vi "Transfer Sample.vi"(8 "error in (no error)":errorcluster, 11 "cRIO-CO2 in":refnum<class "cRIO-CO2.lvclass">) -> (0 "error out":errorcluster, 3 "cRIO-CO2 out":refnum<class "cRIO-CO2.lvclass">)   [LabVIEW 2015, in "cRIO-Carbondioxide.lvlib" / "cRIO-CO2.lvlib" / "cRIO-CO2.lvclass"]
uses:
  cRIO-CO2.lvclass
  cRIO-CO2.lvclass/cRIO-CO2.ctl
  <vilib>/ActorFramework/Time-Delayed Send Message/Time-Delay Override Options.ctl
  Controls/Sample Transfer State Enumerator.ctl
  subs/Sample/Sample.lvclass
  <vilib>/ActorFramework/Message Enqueuer/Message Enqueuer.lvclass/Message Enqueuer.ctl
  subs/Sample/Sample.lvclass/Sample.ctl
  Controls/Sample Transfer Container Enumerator.ctl
  Controls/Vacuum State Enumerator.ctl
  <vilib>/ActorFramework/Message Enqueuer/Enqueue.vi
  State Elapsed Time.vi
  <vilib>/ActorFramework/Message Priority Queue/Priority Enqueue.vi
  Transfer Line Messages/Sample Out Msg/Sample Out Msg.lvclass
panel:
  out "Waveform Chart":ext(graph)
  out "time stamp":timestamp
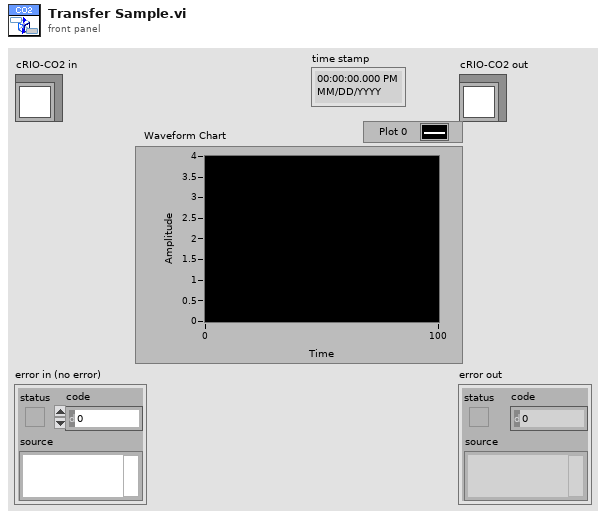
[diagram p1: front panel]
types:
  T1 = typedef "Time-Delay Override Options.ctl" = enum16{"Send next copy now", "Skip next scheduled copy", "Send next copy now and stop all further copies", "Stop all further copies"}
  T2 = typedef "Sample Transfer State Enumerator.ctl" = enum16{"Idle", "Initialize", "Check Containers", "Check Temperatures", "Start Turbo", "Warm Up Containers", "Prepare for purging", "Purge Capillary", "Purge", "Open Containers", "Introduce Sample", "Measure Base Pressure", "Home Syringe", "Start Freezer", "Freeze Target", "Crystalize", "Initiate Stash", "Stash", "Polish", "Stop Freezers", "Push Sample", "Complete", "Abort", "Error", "Undefined"}
  T3 = typedef "Sample Transfer Container Enumerator.ctl" = enum16{"None", "Sample 1", "Sample 2", "Sample 3", "Sample 4", "Sample 5", "Storage 01", "Storage 02", "Storage 03", "Storage 04", "Storage 05", "Storage 06", "Storage 07", "Storage 08", "Storage 09", "Storage 10", "Storage 11", "Storage 12", "Syringe", "Undefined"}
  T4 = typedef "Vacuum State Enumerator.ctl" = enum16{"Pressure Rising", "Plateau", "Pressure Dropping", "Valley", "Low Valley", "Leak", "Unknown"}
  T5 = typedef "cRIO-Carbondioxide.lvlib/cRIO-CO2.lvlib/cRIO-CO2.lvclass/Blowers Heaters Enumerator.ctl" = enum16{"Tank Blower 1", "Tank Blower 2", "Tank Blower 3", "Tank Blower 4", "Syringe Blower", "Syringe Heater", "Piston Heater", "Undefined"}
  T6 = typedef "Sample Container.ctl" = cluster{"Sample In":refnum<k21>, "Sample Name":refnum<k21>, "Ti Cathode":refnum<k21>, "SampleQ":refnum<queue>}
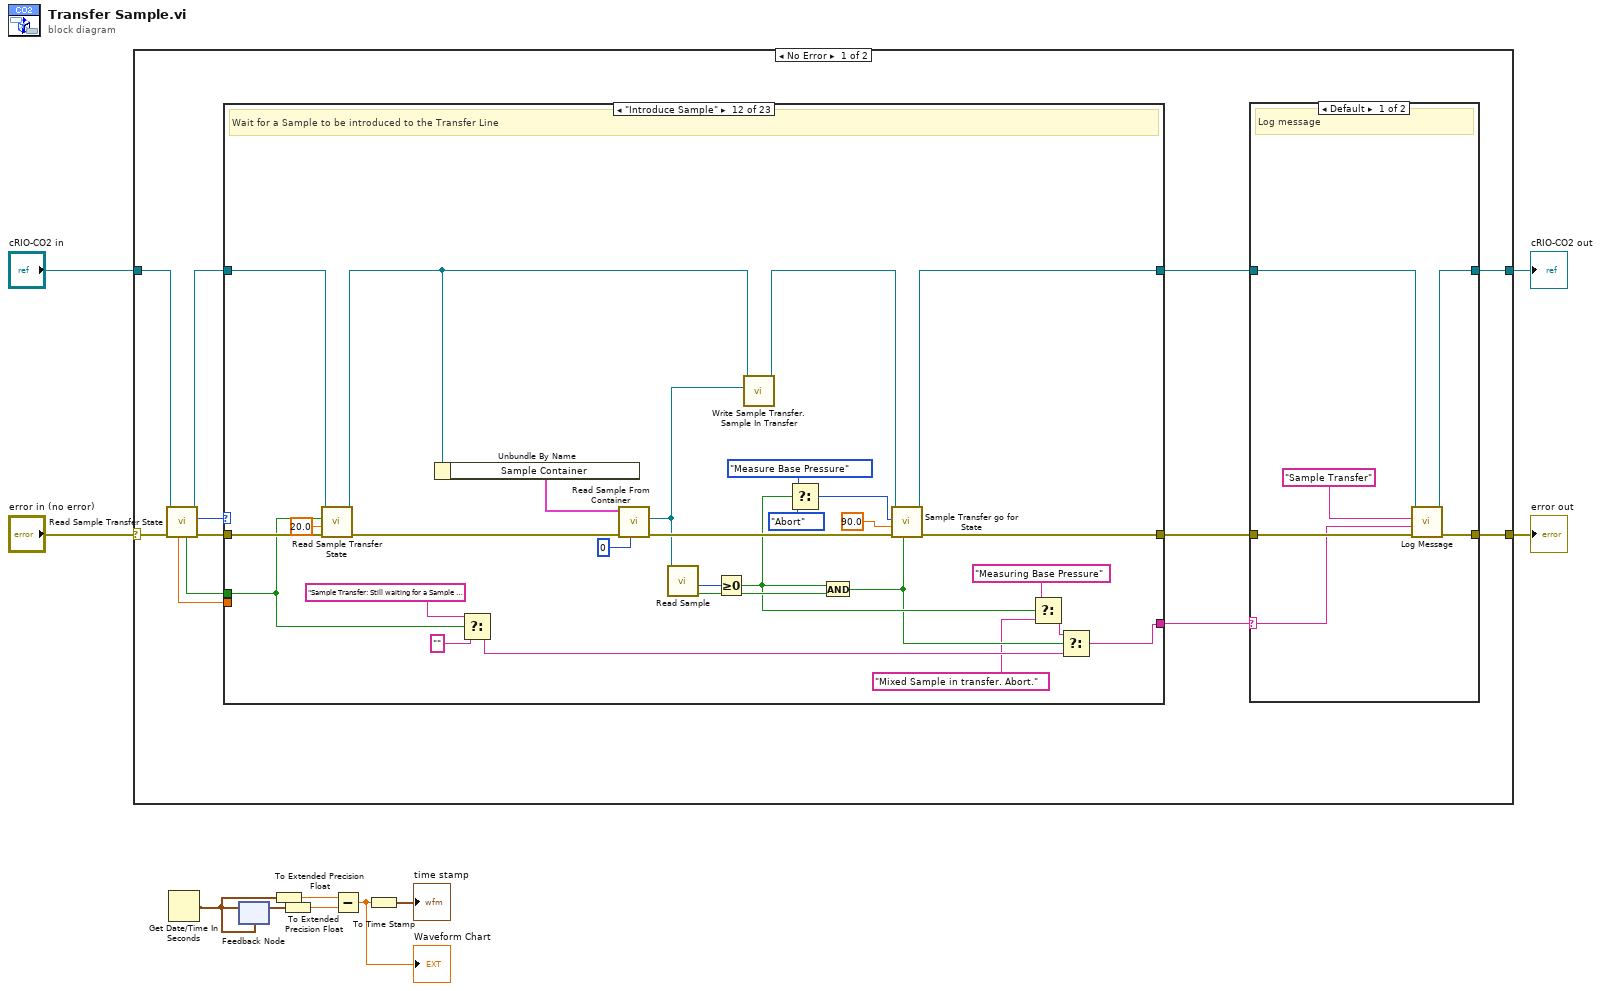
[diagram p0: block diagram]
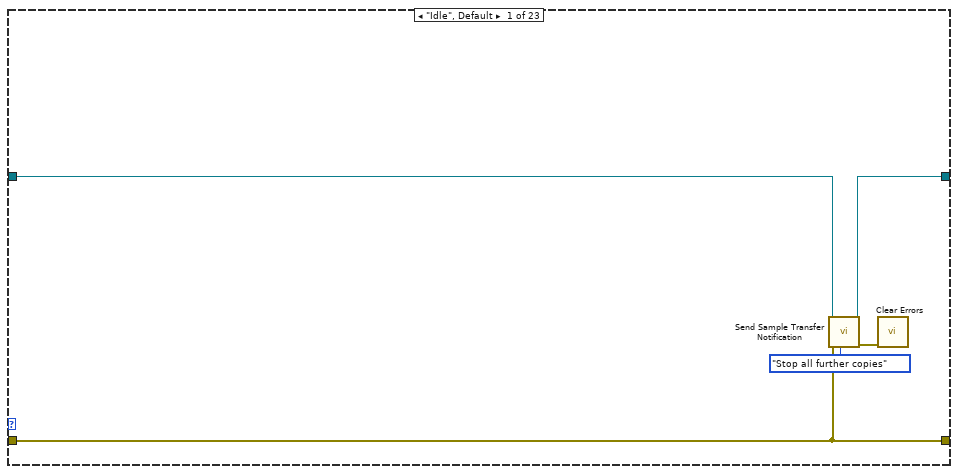
[diagram p3: hidden frame]
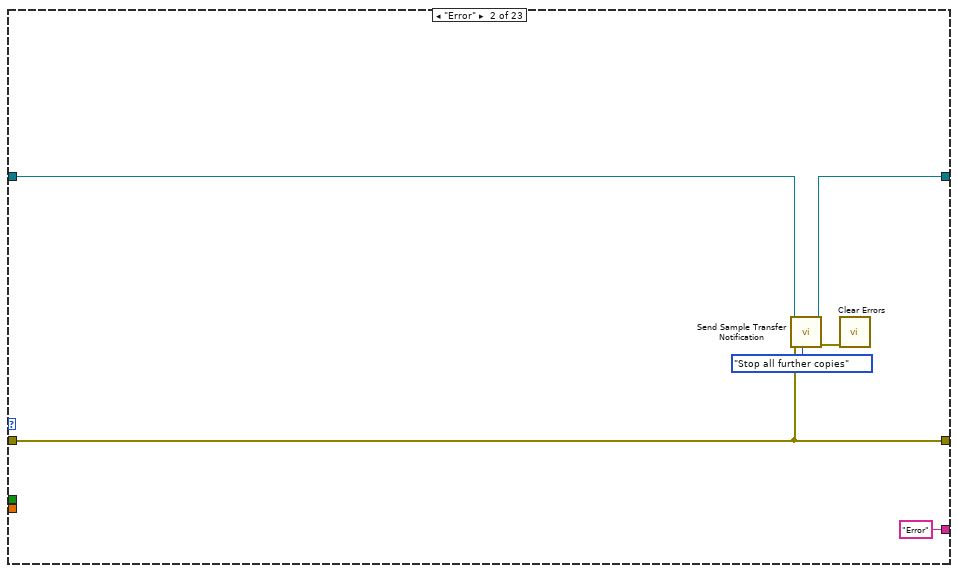
[diagram p4: hidden frame]
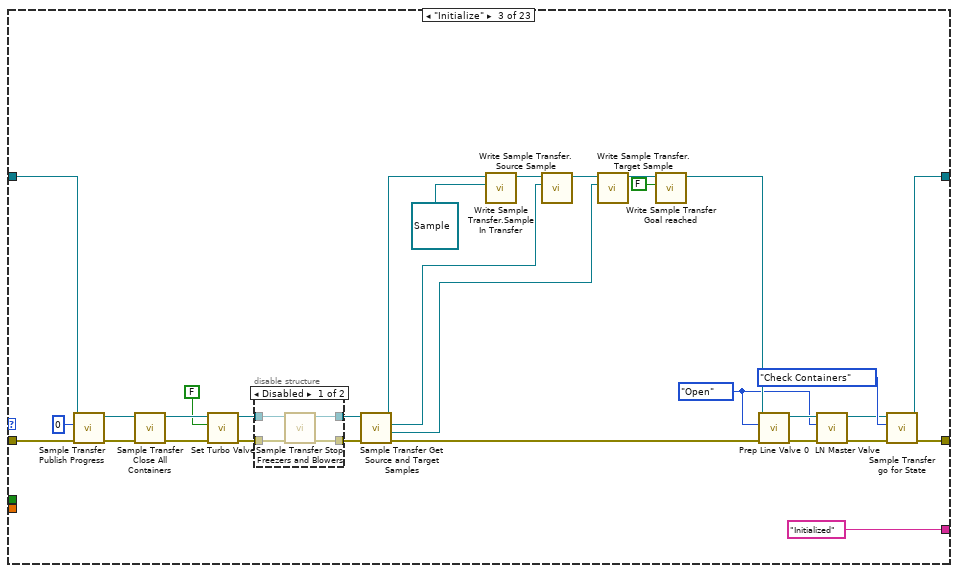
[diagram p5: hidden frame]
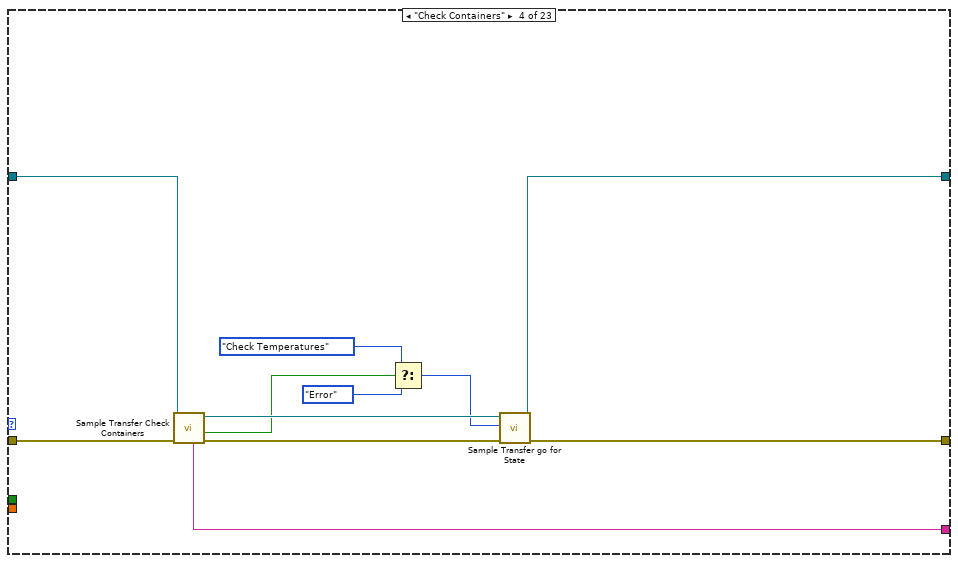
[diagram p7: hidden frame]
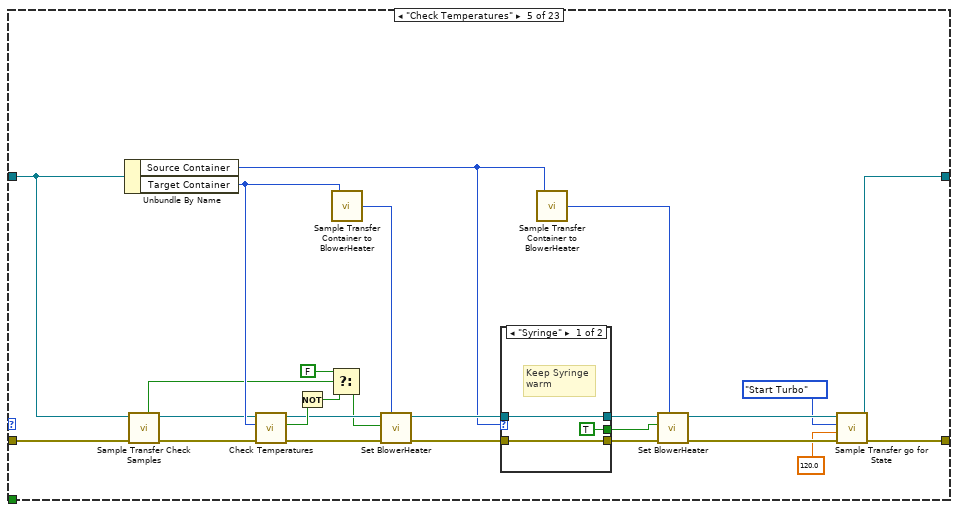
[diagram p8: hidden frame]
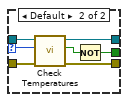
[diagram p9: hidden frame]
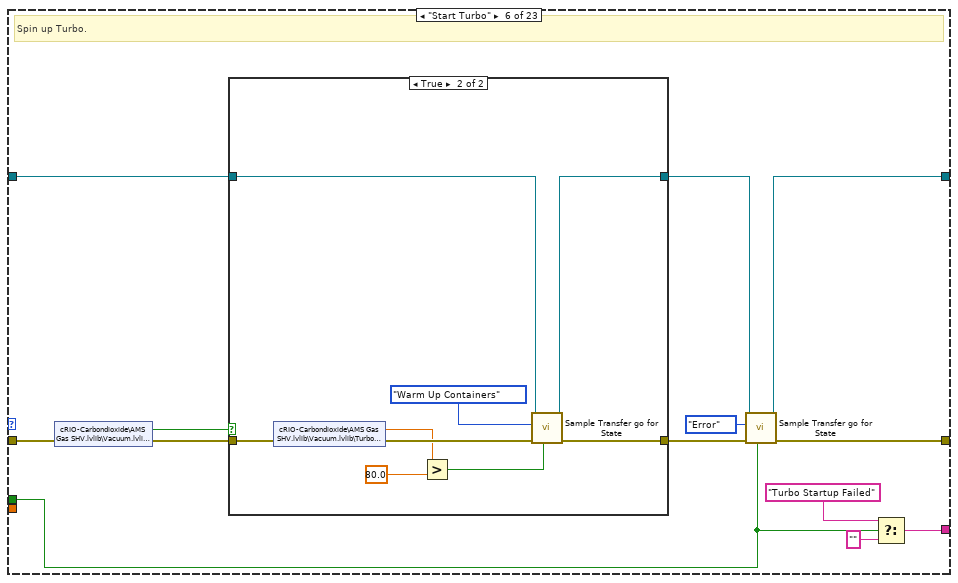
[diagram p10: hidden frame]
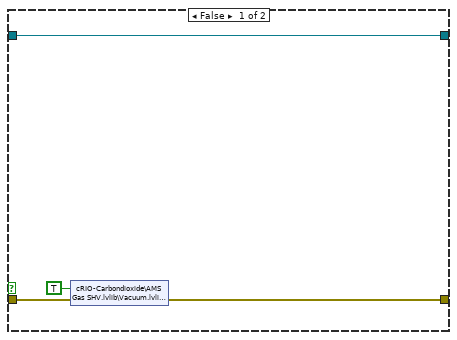
[diagram p11: hidden frame]
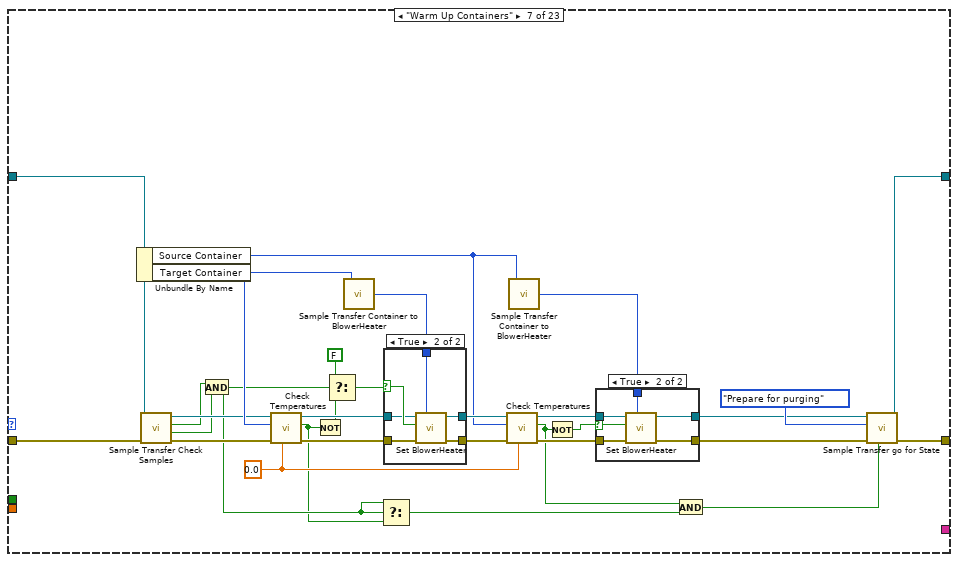
[diagram p12: hidden frame]
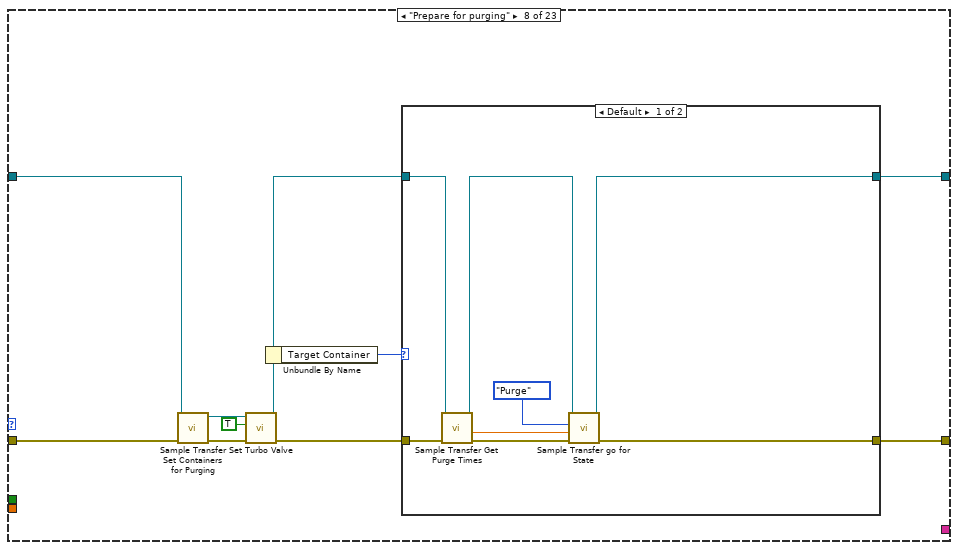
[diagram p15: hidden frame]
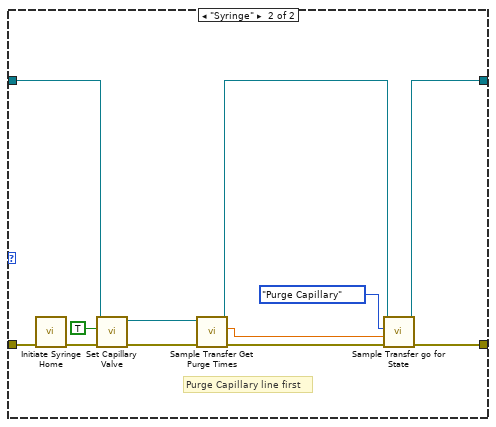
[diagram p16: hidden frame]
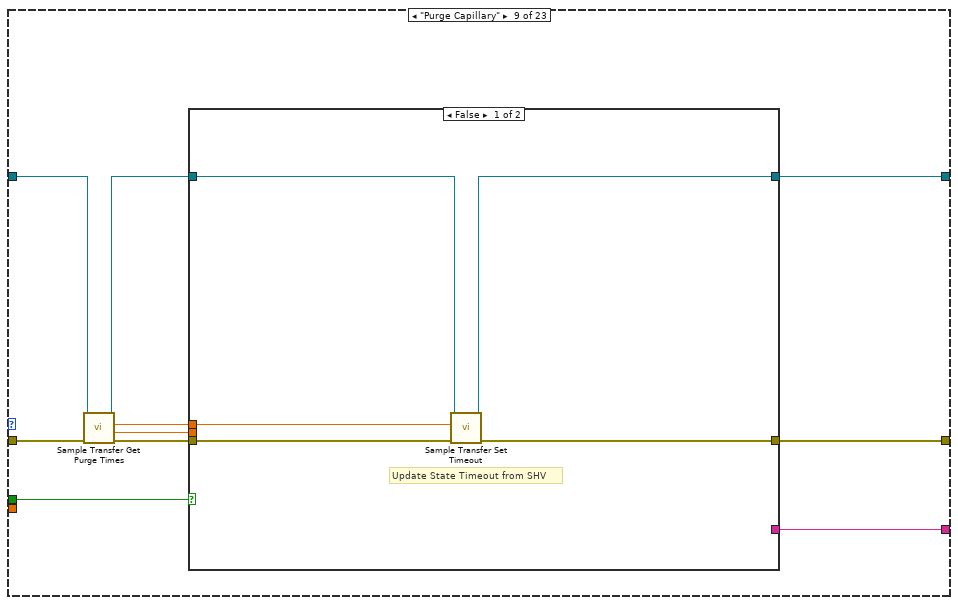
[diagram p17: hidden frame]
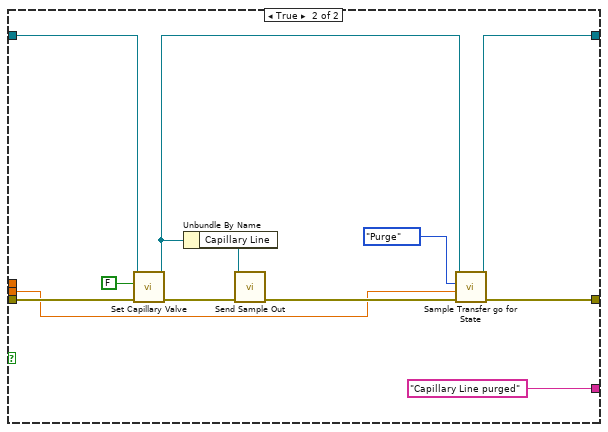
[diagram p18: hidden frame]
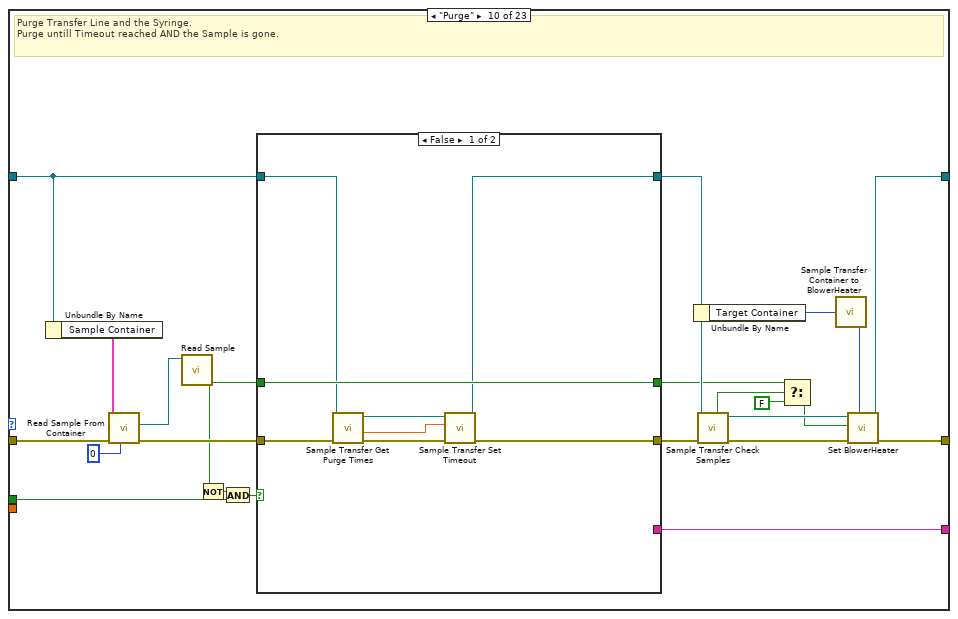
[diagram p19: hidden frame]
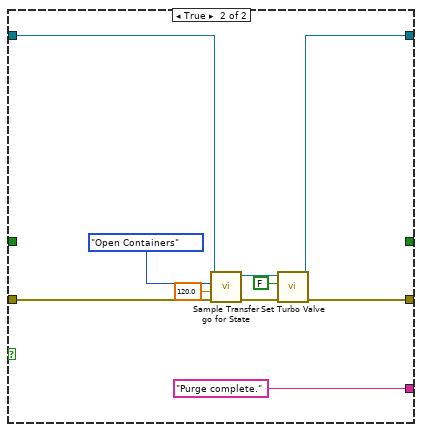
[diagram p20: hidden frame]
diagram:
  n1 = case shown="No Error" "error in (no error)" {
    selector: "error in (no error)" -> [w22 w715]
    tunnel: [w15 w715] -> w9
    tunnel: [w14 w714] -> w7
    tunnel: "cRIO-CO2 in" -> [w21 w714]
    frame No Error {
      n2 = call "Read Sample Transfer State.vi"("error in (no error)"=w22, "cRIO-CO2 in"=w21) -> ("error out"=w20:errorcluster, "Sample Transfer State"=w19:T2, "cRIO-CO2 out"=w18:refnum<class "cRIO-CO2.lvclass">, "Timeout?"=w13:bool, "Elapsed Time (s)"=w11:dbl)  [unwired: 4 in, 1 out]
      n3 = case shown="\"Introduce Sample\"" w19 {
        tunnel: w20 -> [w31 w38 w61 w89 w98 w135 w161 w208 w234 w275 w307 w355 w366 w410 w419 w446 w477 w580 w608 w653 w669 w689 w713]
        tunnel: w18 -> [w34 w37 w72 w88 w100 w136 w163 w202 w232 w276 w303 w353 w365 w413 w421 w440 w481 w578 w612 w652 w668 w680 w711]
        tunnel: [w31 w38 w69 w85 w103 w133 w182 w200 w236 w277 w305 w347 w369 w414 w415 w447 w479 w573 w610 w657 w662 w682 w701] -> w16
        tunnel: [_ "Error" ("String") "Initialized" ("String") w80 _ w126 _ _ w235 w278 "Open Source Container" ("string") w356 w367 "Syringe homed" w423 _ w476 "Initiating Stash" ("String") w607 _ w658 "Complete" ("String") "Sample Transfer Aborted" ("String")] -> w17
        tunnel: w13 -> [_ _ _ _ _ w128 _ _ w238 w261 _ w351 w360 _ _ _ w478 _ w609 w654 _ _ _]
        tunnel: [w33 w39 w60 w86 w104 w131 w181 w199 w237 w263 w301 w348 w368 w412 w416 w448 w480 w571 w611 w656 w660 w681 w702] -> w12
        tunnel: w11 -> [_ _ _ _ _ _ _ _ _ _ _ _ _ _ _ _ _ _ _ _ _ _ _]
        frame "Idle", Default {
          n4 = call "Send Sample Transfer Notification.vi"("notification (Send next copy now)"=Time-Delay_Override_Options."Stop all further copies", "error in (no error)"=w31, "cRIO-CO2 in"=w34) -> ("error out"=w32:errorcluster, "cRIO-CO2 out"=w33:refnum<class "cRIO-CO2.lvclass">)  [unwired: 7 in]
          n5 = call <vilib>:"Clear Errors.vi"("error in (no error)"=w32) -> ()  [unwired: 5 in, 2 out]
        }
        frame "Error" {
          n6 = call "Send Sample Transfer Notification.vi"("notification (Send next copy now)"=Time-Delay_Override_Options."Stop all further copies", "error in (no error)"=w38, "cRIO-CO2 in"=w37) -> ("error out"=w40:errorcluster, "cRIO-CO2 out"=w39:refnum<class "cRIO-CO2.lvclass">)  [unwired: 7 in]
          n7 = call <vilib>:"Clear Errors.vi"("error in (no error)"=w40) -> ()  [unwired: 5 in, 2 out]
        }
        frame "Initialize" {
          w43 = enum16{"Read State", "Open", "Close"}."Open" ("Action (Read State)")
          n8 = call "Sample Transfer Publish Progress.vi"("error in (no error)"=w61, "Progress"=u8 0, "cRIO-CO2 in"=w72) -> ("error out"=w65:errorcluster, "cRIO-CO2 out"=w64:refnum<class "cRIO-CO2.lvclass">)  [unwired: 7 in]
          n9 = call "Sample Transfer Close All Containers.vi"("error in (no error)"=w65, "cRIO-CO2 in"=w64) -> ("error out"=w68:errorcluster, "cRIO-CO2 out"=w67:refnum<class "cRIO-CO2.lvclass">)  [unwired: 8 in]
          n10 = call "Set Turbo Valve.vi"("error in (no error)"=w68, "ON/OFF(OFF)"=FALSE, "cRIO-CO2 in"=w67) -> ("error out"=w62:errorcluster, "cRIO-CO2 out"=w63:refnum<class "cRIO-CO2.lvclass">)  [unwired: 7 in]
          n11 = disable-structure shown="Disabled" {
            disable-tunnel: w63 -> [w76 w77]
            disable-tunnel: w62 -> [w75 w78]
            disable-tunnel: [w74 w78] -> w59
            disable-tunnel: [w73 w77] -> w58
            frame Disabled {
              n12 = call "Sample Transfer Stop Freezers and Blowers.vi"("error in (no error)"=w75, "cRIO-CO2 in"=w76) -> ("error out"=w74:errorcluster, "cRIO-CO2 out"=w73:refnum<class "cRIO-CO2.lvclass">)  [unwired: 8 in]
            }
            frame Enabled {
            }
          }
          n13 = call "Sample Transfer Get Source and Target Samples.vi"("error in (no error)"=w59, "cRIO-CO2 in"=w58) -> ("error out"=w47:errorcluster, "Sample in Target Container"=w53:refnum<class "Sample.lvclass">, "Sample in Source Container"=w54:refnum<class "Sample.lvclass">, "cRIO-CO2 out"=w57:refnum<class "cRIO-CO2.lvclass">)  [unwired: 6 in]
          n14 = call "Write Sample Transfer.Sample In Transfer.vi"("Sample.lvclass"=refnum<class "Sample.lvclass"> refnum ("Sample Transfer.Sample"), "cRIO-CO2 in"=w57) -> ("cRIO-CO2 out"=w55:refnum<class "cRIO-CO2.lvclass">)  [unwired: 9 in]
          n15 = call "Write Sample Transfer.Source Sample.vi"("Sample.lvclass"=w54, "cRIO-CO2 in"=w55) -> ("cRIO-CO2 out"=w56:refnum<class "cRIO-CO2.lvclass">)  [unwired: 9 in]
          n16 = call "Write Sample Transfer.Target Sample.vi"("Sample.lvclass"=w53, "cRIO-CO2 in"=w56) -> ("cRIO-CO2 out"=w52:refnum<class "cRIO-CO2.lvclass">)  [unwired: 9 in]
          n17 = call "Write Sample Transfer Goal reached.vi"("Goal reached"=FALSE, "cRIO-CO2 in"=w52) -> ("cRIO-CO2 out"=w45:refnum<class "cRIO-CO2.lvclass">)  [unwired: 9 in]
          n18 = call "Prep Line Valve 0.vi"("error in (no error)"=w47, "Action (Read State)"=w43, "cRIO-CO2 in"=w45) -> ("error out"=w46:errorcluster, "cRIO-CO2 out"=w44:refnum<class "cRIO-CO2.lvclass">)  [unwired: 6 in, 1 out]
          n19 = call "LN Master Valve.vi"("error in (no error)"=w46, "Action (Read State)"=w43, "cRIO-CO2 in"=w44) -> ("error out"=w50:errorcluster, "cRIO-CO2 out"=w48:refnum<class "cRIO-CO2.lvclass">)  [unwired: 6 in, 1 out]
          n20 = call "Sample Transfer go for State.vi"("error in (no error)"=w50, "Sample Transfer State"=Sample_Transfer_State_Enumerator."Check Containers", "cRIO-CO2 in"=w48) -> ("error out"=w69:errorcluster, "cRIO-CO2 out"=w60:refnum<class "cRIO-CO2.lvclass">)  [unwired: 7 in]
        }
        frame "Check Containers" {
          n21 = call "Sample Transfer Check Containers.vi"("error in (no error)"=w89, "cRIO-CO2 in"=w88) -> ("error out"=w87:errorcluster, "Valid Containers?"=w83:bool, "cRIO-CO2 out"=w84:refnum<class "cRIO-CO2.lvclass">, "Message"=w80:string)  [unwired: 6 in]
          n22 = Select(t=Sample_Transfer_State_Enumerator."Check Temperatures", s=w83, f=Sample_Transfer_State_Enumerator."Error" ("Sample Transfer State")) -> (s? t:f=w82:T2)
          n23 = call "Sample Transfer go for State.vi"("error in (no error)"=w87, "Sample Transfer State"=w82, "cRIO-CO2 in"=w84) -> ("error out"=w85:errorcluster, "cRIO-CO2 out"=w86:refnum<class "cRIO-CO2.lvclass">)  [unwired: 7 in]
        }
        frame "Check Temperatures" {
          n24 = Unbundle By Name(w100) -> ("Source Container"=w112:T3, "Target Container"=w101:T3)
          n25 = call "Sample Transfer Check Samples.vi"("error in (no error)"=w98, "cRIO-CO2 in"=w100) -> ("error out"=w97:errorcluster, "cRIO-CO2 out"=w99:refnum<class "cRIO-CO2.lvclass">, "Same Sample AND Target not Empty"=w90:bool)  [unwired: 5 in, 2 out]
          n26 = call "Check Temperatures.vi"("error in (no error)"=w97, "Container"=w101, "cRIO-CO2 in"=w99) -> ("error out"=w96:errorcluster, "In Range?"=w95:bool, "cRIO-CO2 out"=w94:refnum<class "cRIO-CO2.lvclass">)  [unwired: 6 in]
          n27 = Not(x=w95) -> (.not. x?=w93:bool)
          n28 = Select(t=FALSE, s=w90, f=w93) -> (s? t:f=w91:bool)
          n29 = call "Sample Transfer Container to BlowerHeater.vi"("Container"=w101) -> ("Blower/Heater"=w113:T5)  [unwired: 4 in]
          n30 = call "Set BlowerHeater.vi"("Blower/Heater"=w113, "error in (no error)"=w96, "ON/OFF (OFF)"=w91, "cRIO-CO2 in"=w94) -> ("error out"=w115:errorcluster, "cRIO-CO2 out"=w114:refnum<class "cRIO-CO2.lvclass">)  [unwired: 6 in]
          n31 = case shown="\"Syringe\"" w112 {
            selector: w112 -> [_ w123]
            tunnel: w115 -> [w118 w125]
            tunnel: w114 -> [w116 w124]
            tunnel: [w118 w122] -> w111
            tunnel: [w116 w121] -> w110
            tunnel: [TRUE w119] -> w109
            frame "Syringe" {
              # "Keep Syringe\nwarm"
            }
            frame Default {
              n32 = call "Check Temperatures.vi"("error in (no error)"=w125, "Container"=w123, "cRIO-CO2 in"=w124) -> ("error out"=w122:errorcluster, "In Range?"=w120:bool, "cRIO-CO2 out"=w121:refnum<class "cRIO-CO2.lvclass">)  [unwired: 6 in]
              n33 = Not(x=w120) -> (.not. x?=w119:bool)
            }
          }
          n34 = call "Sample Transfer Container to BlowerHeater.vi"("Container"=w112) -> ("Blower/Heater"=w108:T5)  [unwired: 4 in]
          n35 = call "Set BlowerHeater.vi"("Blower/Heater"=w108, "error in (no error)"=w111, "ON/OFF (OFF)"=w109, "cRIO-CO2 in"=w110) -> ("error out"=w107:errorcluster, "cRIO-CO2 out"=w106:refnum<class "cRIO-CO2.lvclass">)  [unwired: 6 in]
          n36 = call "Sample Transfer go for State.vi"("error in (no error)"=w107, "State Timeout (Inf=no timeout )"=120.0, "Sample Transfer State"=Sample_Transfer_State_Enumerator."Start Turbo", "cRIO-CO2 in"=w106) -> ("error out"=w103:errorcluster, "cRIO-CO2 out"=w104:refnum<class "cRIO-CO2.lvclass">)  [unwired: 6 in]
        }
        frame "Start Turbo" {
          # "Spin up Turbo."
          n37 = shared-variable "cRIO-Carbondioxide\\AMS Gas SHV.lvlib\\Vacuum.lvlib\\Turbo ON"(error in=w135) -> (w137:bool, error out=w138:errorcluster)
          n38 = case shown="True" w137 {
            tunnel: w138 -> [w141 w151]
            tunnel: w136 -> [w142 w149]
            tunnel: [w142 w148] -> w132
            tunnel: [w140 w145] -> w134
            frame False {
              n39 = shared-variable "cRIO-Carbondioxide\\AMS Gas SHV.lvlib\\Vacuum.lvlib\\Turbo ON"(TRUE ("Turbo ON"), error in=w141) -> (error out=w140:errorcluster)
            }
            frame True {
              n40 = shared-variable "cRIO-Carbondioxide\\AMS Gas SHV.lvlib\\Vacuum.lvlib\\Turbo Speed"(error in=w151) -> (w147:dbl, error out=w150:errorcluster)
              n41 = Greater?(x=w147, y=80.0) -> (0:w143:bool)
              n42 = call "Sample Transfer go for State.vi"("Really? (T)"=w143, "error in (no error)"=w150, "Sample Transfer State"=Sample_Transfer_State_Enumerator."Warm Up Containers", "cRIO-CO2 in"=w149) -> ("error out"=w145:errorcluster, "cRIO-CO2 out"=w148:refnum<class "cRIO-CO2.lvclass">)  [unwired: 6 in]
            }
          }
          n43 = call "Sample Transfer go for State.vi"("Really? (T)"=w128, "error in (no error)"=w134, "Sample Transfer State"=Sample_Transfer_State_Enumerator."Error", "cRIO-CO2 in"=w132) -> ("error out"=w133:errorcluster, "cRIO-CO2 out"=w131:refnum<class "cRIO-CO2.lvclass">)  [unwired: 6 in]
          n44 = Select(t="Turbo Startup Failed" ("String"), s=w128, f="") -> (s? t:f=w126:string)
        }
        frame "Warm Up Containers" {
          w165 = 0.0 ("lower limit (10C)")
          n45 = Unbundle By Name(w163) -> ("Source Container"=w173:T3, "Target Container"=w164:T3)
          n46 = call "Sample Transfer Check Samples.vi"("error in (no error)"=w161, "cRIO-CO2 in"=w163) -> ("error out"=w160:errorcluster, "Target not Empty"=w159:bool, "Same Sample in Source and Target"=w158:bool, "cRIO-CO2 out"=w162:refnum<class "cRIO-CO2.lvclass">)  [unwired: 5 in, 1 out]
          n47 = And(x=w158, y=w159) -> (x .and. y?=w153:bool)
          n48 = call "Check Temperatures.vi"("lower limit (10C)"=w165, "error in (no error)"=w160, "Container"=w164, "cRIO-CO2 in"=w162) -> ("error out"=w178:errorcluster, "In Range?"=w152:bool, "cRIO-CO2 out"=w177:refnum<class "cRIO-CO2.lvclass">)  [unwired: 5 in]
          n49 = Not(x=w152) -> (.not. x?=w157:bool)
          n50 = Select(t=FALSE, s=w153, f=w157) -> (s? t:f=w156:bool)
          n51 = call "Sample Transfer Container to BlowerHeater.vi"("Container"=w164) -> ("Blower/Heater"=w174:T5)  [unwired: 4 in]
          n52 = Select(t=w153, s=w153, f=w152) -> (s? t:f=w154:bool)
          n53 = case shown="True" w156 {
            selector: w156 -> [_ w197]
            tunnel: w178 -> [w191 w198]
            tunnel: w177 -> [w192 w196]
            tunnel: [w191 w195] -> w176
            tunnel: [w192 w194] -> w175
            tunnel: w174 -> [_ w193]
            frame False {
            }
            frame True {
              n54 = call "Set BlowerHeater.vi"("Blower/Heater"=w193, "error in (no error)"=w198, "ON/OFF (OFF)"=w197, "cRIO-CO2 in"=w196) -> ("error out"=w195:errorcluster, "cRIO-CO2 out"=w194:refnum<class "cRIO-CO2.lvclass">)  [unwired: 6 in]
            }
          }
          n55 = call "Check Temperatures.vi"("lower limit (10C)"=w165, "error in (no error)"=w176, "Container"=w173, "cRIO-CO2 in"=w175) -> ("error out"=w172:errorcluster, "In Range?"=w168:bool, "cRIO-CO2 out"=w171:refnum<class "cRIO-CO2.lvclass">)  [unwired: 5 in]
          n56 = call "Sample Transfer Container to BlowerHeater.vi"("Container"=w173) -> ("Blower/Heater"=w169:T5)  [unwired: 4 in]
          n57 = Not(x=w168) -> (.not. x?=w170:bool)
          n58 = case shown="True" w170 {
            selector: w170 -> [_ w188]
            tunnel: w172 -> [w183 w190]
            tunnel: w171 -> [w184 w189]
            tunnel: w169 -> [_ w187]
            tunnel: [w183 w186] -> w167
            tunnel: [w184 w185] -> w166
            frame False {
            }
            frame True {
              n59 = call "Set BlowerHeater.vi"("Blower/Heater"=w187, "error in (no error)"=w190, "ON/OFF (OFF)"=w188, "cRIO-CO2 in"=w189) -> ("error out"=w186:errorcluster, "cRIO-CO2 out"=w185:refnum<class "cRIO-CO2.lvclass">)  [unwired: 6 in]
            }
          }
          n60 = And(x=w168, y=w154) -> (x .and. y?=w179:bool)
          n61 = call "Sample Transfer go for State.vi"("Really? (T)"=w179, "error in (no error)"=w167, "Sample Transfer State"=Sample_Transfer_State_Enumerator."Prepare for purging", "cRIO-CO2 in"=w166) -> ("error out"=w182:errorcluster, "cRIO-CO2 out"=w181:refnum<class "cRIO-CO2.lvclass">)  [unwired: 6 in]
        }
        frame "Prepare for purging" {
          n62 = call "Sample Transfer Set Containers for Purging.vi"("error in (no error)"=w208, "cRIO-CO2 in"=w202) -> ("error out"=w206:errorcluster, "cRIO-CO2 out"=w205:refnum<class "cRIO-CO2.lvclass">)  [unwired: 8 in]
          n63 = call "Set Turbo Valve.vi"("error in (no error)"=w206, "ON/OFF(OFF)"=TRUE, "cRIO-CO2 in"=w205) -> ("error out"=w204:errorcluster, "cRIO-CO2 out"=w201:refnum<class "cRIO-CO2.lvclass">)  [unwired: 7 in]
          n64 = Unbundle By Name(w201) -> ("Target Container"=w203:T3)
          n65 = case shown="Default" w203 {
            tunnel: w204 -> [w213 w224]
            tunnel: [w215 w228] -> w200
            tunnel: w201 -> [w211 w225]
            tunnel: [w214 w227] -> w199
            frame Default {
              n66 = call "Sample Transfer Get Purge Times.vi"("error in (no error)"=w213, "cRIO-CO2 in"=w211) -> ("error out"=w212:errorcluster, "Purge Time (sec)"=w209:dbl, "cRIO-CO2 out"=w210:refnum<class "cRIO-CO2.lvclass">)  [unwired: 6 in, 1 out]
              n67 = call "Sample Transfer go for State.vi"("error in (no error)"=w212, "State Timeout (Inf=no timeout )"=w209, "Sample Transfer State"=Sample_Transfer_State_Enumerator."Purge", "cRIO-CO2 in"=w210) -> ("error out"=w215:errorcluster, "cRIO-CO2 out"=w214:refnum<class "cRIO-CO2.lvclass">)  [unwired: 6 in]
            }
            frame "Syringe" {
              # "Purge Capillary line first"
              n68 = call "Initiate Syringe Home.vi"("error in (no error)"=w224) -> ("error out"=w223:errorcluster)  [unwired: 10 in]
              n69 = call "Set Capillary Valve.vi"("error in (no error)"=w223, "ON/OFF(OFF)"=TRUE ("Syringe-Capillary Valve HV315"), "cRIO-CO2 in"=w225) -> ("error out"=w221:errorcluster, "cRIO-CO2 out"=w220:refnum<class "cRIO-CO2.lvclass">)  [unwired: 7 in]
              n70 = call "Sample Transfer Get Purge Times.vi"("error in (no error)"=w221, "cRIO-CO2 in"=w220) -> ("error out"=w218:errorcluster, "Purge Capillary Time (sec)"=w217:dbl, "cRIO-CO2 out"=w219:refnum<class "cRIO-CO2.lvclass">)  [unwired: 6 in, 1 out]
              n71 = call "Sample Transfer go for State.vi"("error in (no error)"=w218, "State Timeout (Inf=no timeout )"=w217, "Sample Transfer State"=Sample_Transfer_State_Enumerator."Purge Capillary", "cRIO-CO2 in"=w219) -> ("error out"=w228:errorcluster, "cRIO-CO2 out"=w227:refnum<class "cRIO-CO2.lvclass">)  [unwired: 6 in]
            }
          }
        }
        frame "Purge Capillary" {
          n72 = call "Sample Transfer Get Purge Times.vi"("error in (no error)"=w234, "cRIO-CO2 in"=w232) -> ("error out"=w233:errorcluster, "Purge Time (sec)"=w230:dbl, "Purge Capillary Time (sec)"=w229:dbl, "cRIO-CO2 out"=w231:refnum<class "cRIO-CO2.lvclass">)  [unwired: 6 in]
          n73 = case shown="False" w238 {
            tunnel: w233 -> [w243 w252]
            tunnel: w231 -> [w240 w250]
            tunnel: [w239 w255] -> w237
            tunnel: [w242 w254] -> w236
            tunnel: [_ "Capillary Line purged" ("String")] -> w235
            tunnel: w230 -> [_ w244]
            tunnel: w229 -> [w241 _]
            frame False {
              # "Update State Timeout from SHV"
              n74 = call "Sample Transfer Set Timeout.vi"("error in (no error)"=w243, "Sample Transfer.State Timeout (0)"=w241, "cRIO-CO2 in"=w240) -> ("error out"=w242:errorcluster, "cRIO-CO2 out"=w239:refnum<class "cRIO-CO2.lvclass">)  [unwired: 7 in]
            }
            frame True {
              n75 = call "Set Capillary Valve.vi"("error in (no error)"=w252, "ON/OFF(OFF)"=FALSE ("Syringe-Capillary Valve HV315"), "cRIO-CO2 in"=w250) -> ("error out"=w249:errorcluster, "cRIO-CO2 out"=w245:refnum<class "cRIO-CO2.lvclass">)  [unwired: 7 in]
              n76 = Unbundle By Name(w245) -> ("Capillary Line"=w248:refnum<class "Message Enqueuer.lvclass">)
              n77 = call "Send Sample Out.vi"("error in (no error)"=w249, "Message Enqueuer"=w248) -> ("error out"=w246:errorcluster)  [unwired: 8 in, 1 out]
              n78 = call "Sample Transfer go for State.vi"("error in (no error)"=w246, "State Timeout (Inf=no timeout )"=w244, "Sample Transfer State"=Sample_Transfer_State_Enumerator."Purge", "cRIO-CO2 in"=w245) -> ("error out"=w254:errorcluster, "cRIO-CO2 out"=w255:refnum<class "cRIO-CO2.lvclass">)  [unwired: 6 in]
            }
          }
        }
        frame "Purge" {
          # "Purge Transfer Line and the Syringe.\nPurge untill Timeout reached AND the Sample is gone."
          n79 = Unbundle By Name(w276) -> ("Sample Container"=w272:T6)
          n80 = call "Read Sample From Container.vi"("Queue timeout in ms (-1)"=0, "error in (no error)"=w275, "Container"=w272) -> ("error out"=w271:errorcluster, "Sample out"=w264:refnum<class "Sample.lvclass">)  [unwired: 4 in, 3 out]
          n81 = call "Read Sample.vi"("Sample in"=w264) -> ("Sample In"=w259:bool)  [unwired: 6 in, 4 out]
          n82 = Not(x=w259) -> (.not. x?=w258:bool)
          n83 = And(x=w258, y=w261) -> (x .and. y?=w260:bool)
          n84 = case shown="False" w260 {
            tunnel: [_ "Purge complete." ("f")] -> w278
            tunnel: w276 -> [w284 w296]
            tunnel: w271 -> [w285 w293]
            tunnel: [w282 w287] -> w269
            tunnel: w259 -> [w286 _]
            tunnel: [w280 w291] -> w262
            tunnel: [w286 _] -> w257
            frame False {
              n85 = call "Sample Transfer Get Purge Times.vi"("error in (no error)"=w285, "cRIO-CO2 in"=w284) -> ("error out"=w283:errorcluster, "Purge Time (sec)"=w279:dbl, "cRIO-CO2 out"=w281:refnum<class "cRIO-CO2.lvclass">)  [unwired: 6 in, 1 out]
              n86 = call "Sample Transfer Set Timeout.vi"("error in (no error)"=w283, "Sample Transfer.State Timeout (0)"=w279, "cRIO-CO2 in"=w281) -> ("error out"=w282:errorcluster, "cRIO-CO2 out"=w280:refnum<class "cRIO-CO2.lvclass">)  [unwired: 7 in]
            }
            frame True {
              n87 = call "Sample Transfer go for State.vi"("error in (no error)"=w293, "State Timeout (Inf=no timeout )"=120.0, "Sample Transfer State"=Sample_Transfer_State_Enumerator."Open Containers", "cRIO-CO2 in"=w296) -> ("error out"=w294:errorcluster, "cRIO-CO2 out"=w292:refnum<class "cRIO-CO2.lvclass">)  [unwired: 6 in]
              n88 = call "Set Turbo Valve.vi"("error in (no error)"=w294, "ON/OFF(OFF)"=FALSE, "cRIO-CO2 in"=w292) -> ("error out"=w287:errorcluster, "cRIO-CO2 out"=w291:refnum<class "cRIO-CO2.lvclass">)  [unwired: 7 in]
            }
          }
          n89 = Unbundle By Name(w262) -> ("Target Container"=w274:T3)
          n90 = call "Sample Transfer Check Samples.vi"("error in (no error)"=w269, "cRIO-CO2 in"=w262) -> ("error out"=w268:errorcluster, "cRIO-CO2 out"=w267:refnum<class "cRIO-CO2.lvclass">, "Same Sample AND Target not Empty"=w265:bool)  [unwired: 5 in, 2 out]
          n91 = Select(t=w257, s=w265, f=FALSE ("t")) -> (s? t:f=w266:bool)
          n92 = call "Sample Transfer Container to BlowerHeater.vi"("Container"=w274) -> ("Blower/Heater"=w273:T5)  [unwired: 4 in]
          n93 = call "Set BlowerHeater.vi"("Blower/Heater"=w273, "error in (no error)"=w268, "ON/OFF (OFF)"=w266, "cRIO-CO2 in"=w267) -> ("error out"=w277:errorcluster, "cRIO-CO2 out"=w263:refnum<class "cRIO-CO2.lvclass">)  [unwired: 6 in]
        }
        frame "Open Containers" {
          n94 = Unbundle By Name(w303) -> ("Target Container"=w299:T3, "Source Container"=w300:T3)
          n95 = case shown="Default" w300 {
            selector: w300 -> [w309 _]
            tunnel: w307 -> [w310 w330]
            tunnel: [w317 w330] -> w297
            tunnel: w303 -> [w318 w331]
            tunnel: [w312 w331] -> w302
            tunnel: w299 -> [_ _]
            frame Default {
              n96 = case shown="\"Syringe\"" w309 {
                tunnel: w310 -> [w319 w321]
                tunnel: [w319 w320] -> w308
                frame "None", Default {
                }
                frame "Syringe" {
                  n97 = call "Initiate Syringe Home.vi"("error in (no error)"=w321) -> ("error out"=w320:errorcluster)  [unwired: 10 in]
                }
              }
              n98 = call "Sample Transfer Open Source Container.vi"("error in (no error)"=w308, "cRIO-CO2 in"=w318) -> ("error out"=w314:errorcluster, "cRIO-CO2 out"=w316:refnum<class "cRIO-CO2.lvclass">)  [unwired: 8 in]
              n99 = call "Sample Transfer Check Samples.vi"("error in (no error)"=w314, "cRIO-CO2 in"=w316) -> ("error out"=w313:errorcluster, "cRIO-CO2 out"=w315:refnum<class "cRIO-CO2.lvclass">, "Same Sample AND Target not Empty"=w311:bool)  [unwired: 5 in, 2 out]
              n100 = case shown="True" w311 {
                tunnel: [w325 w326] -> w317
                tunnel: w315 -> [w324 w328]
                tunnel: w313 -> [w323 w329]
                tunnel: [w322 w327] -> w312
                frame False {
                  n101 = call "Sample Transfer Open Target Container.vi"("error in (no error)"=w323, "cRIO-CO2 in"=w324) -> ("error out"=w325:errorcluster, "cRIO-CO2 out"=w322:refnum<class "cRIO-CO2.lvclass">)  [unwired: 8 in]
                }
                frame True {
                  # "Keep closed"
                  # "Same Sample\nAND\nTarget not Empty"
                  n102 = call "Sample Transfer Close Target Container.vi"("error in (no error)"=w329, "cRIO-CO2 in"=w328) -> ("error out"=w326:errorcluster, "cRIO-CO2 out"=w327:refnum<class "cRIO-CO2.lvclass">)  [unwired: 8 in]
                }
              }
            }
            frame "Sample 1".."Sample 5" {
              # "Sample Container is supposed\nto be open by now."
              # "Source is the Sample Line"
            }
          }
          n103 = call "Sample Transfer go for State.vi"("error in (no error)"=w297, "State Timeout (Inf=no timeout )"=120.0, "Sample Transfer State"=Sample_Transfer_State_Enumerator."Introduce Sample", "cRIO-CO2 in"=w302) -> ("error out"=w305:errorcluster, "cRIO-CO2 out"=w301:refnum<class "cRIO-CO2.lvclass">)  [unwired: 6 in]
        }
        frame "Introduce Sample" {
          # "Wait for a Sample to be introduced to the Transfer Line"
          n104 = call "Read Sample Transfer State.vi"("error in (no error)"=w355, "State Timeout (Inf)"=20.0, "Reinit Timer (F)"=w351, "cRIO-CO2 in"=w353) -> ("error out"=w354:errorcluster, "cRIO-CO2 out"=w334:refnum<class "cRIO-CO2.lvclass">)  [unwired: 2 in, 4 out]
          n105 = Unbundle By Name(w334) -> ("Sample Container"=w344:T6)
          n106 = Select(t="Sample Transfer: Still waiting for a Sample to be introduced to the Transfer Line.", s=w351, f="") -> (s? t:f=w340:string)
          n107 = call "Read Sample From Container.vi"("Queue timeout in ms (-1)"=0, "error in (no error)"=w354, "Container"=w344) -> ("error out"=w359:errorcluster, "Sample out"=w345:refnum<class "Sample.lvclass">)  [unwired: 4 in, 3 out]
          n108 = call "Read Sample.vi"("Sample in"=w345) -> ("Sample In"=w358:bool, "Ti Cathode"=w357:i8)  [unwired: 6 in, 3 out]
          n109 = Greater Or Equal To 0?(x=w357) -> (x >= 0?=w337:bool)
          n110 = call "Write Sample Transfer.Sample In Transfer.vi"("Sample.lvclass"=w345, "cRIO-CO2 in"=w334) -> ("cRIO-CO2 out"=w346:refnum<class "cRIO-CO2.lvclass">)  [unwired: 9 in]
          n111 = Select(t=Sample_Transfer_State_Enumerator."Measure Base Pressure" ("Sample Transfer State"), s=w337, f=Sample_Transfer_State_Enumerator."Abort") -> (s? t:f=w332:T2)
          n112 = And(x=w337, y=w358) -> (x .and. y?=w336:bool)
          n113 = call "Sample Transfer go for State.vi"("Really? (T)"=w336, "error in (no error)"=w359, "State Timeout (Inf=no timeout )"=90.0, "Sample Transfer State"=w332, "cRIO-CO2 in"=w346) -> ("error out"=w347:errorcluster, "cRIO-CO2 out"=w348:refnum<class "cRIO-CO2.lvclass">)  [unwired: 5 in]
          n114 = Select(t="Measuring Base Pressure" ("string"), s=w337, f="Mixed Sample in transfer. Abort.") -> (s? t:f=w338:string)
          n115 = Select(t=w338, s=w336, f=w340) -> (s? t:f=w356:string)
        }
        frame "Measure Base Pressure" {
          n116 = call "Preview Vacuum State.vi"("error in (no error)"=w366, "cRIO-CO2 in"=w365) -> ("error out"=w363:errorcluster, "State"=w361:T4, "Pressure (mBar)"=w362:dbl, "cRIO-CO2 out"=w364:refnum<class "cRIO-CO2.lvclass">)  [unwired: 3 in, 3 out]
          n117 = case shown="\"Plateau\"" w361 {
            tunnel: [w377 w402] -> w369
            tunnel: w364 -> [w376 w394]
            tunnel: [w375 w401] -> w368
            tunnel: w363 -> [w378 w397]
            tunnel: [w373 w384] -> w367
            tunnel: w362 -> [_ w388]
            tunnel: w360 -> [w372 _]
            frame "Pressure Rising", Default {
              n118 = call "Sample Transfer go for State.vi"("Really? (T)"=w372, "error in (no error)"=w378, "Sample Transfer State"=Sample_Transfer_State_Enumerator."Complete", "cRIO-CO2 in"=w376) -> ("error out"=w377:errorcluster, "cRIO-CO2 out"=w375:refnum<class "cRIO-CO2.lvclass">)  [unwired: 6 in]
              n119 = Select(t="Measuring Base Pressure timed out. No Sample in Transfer. -> Complete!", s=w372, f="") -> (s? t:f=w373:string)
            }
            frame "Plateau" {
              # "If Sample pressure is too low,\nreset target to None to \ndisable further Push"
              n120 = Bundle By Name(cluster=w394, "Base Pressure"=w388) -> (w393:refnum<class "cRIO-CO2.lvclass">)
              n121 = call "Read Sample Transfer.Sample In Transfer.vi"("cRIO-CO2 in"=w393) -> ("Sample.lvclass"=w395:refnum<class "Sample.lvclass">, "cRIO-CO2 out"=w392:refnum<class "cRIO-CO2.lvclass">)  [unwired: 9 in]
              n122 = Unbundle By Name(w392) -> ("Target Container"=w383:T3)
              n123 = call "Read Sample.vi"("Sample in"=w395) -> ("Name"=w398:string)  [unwired: 6 in, 4 out]
              n124 = case shown="\"Syringe\"" w383 {
                tunnel: [Sample_Transfer_State_Enumerator."Start Freezer" ("Sample Transfer State") Sample_Transfer_State_Enumerator."Home Syringe" ("Sample Transfer State")] -> w391
                tunnel: w397 -> [w403 w406]
                tunnel: [w403 w405] -> w396
                frame Default {
                }
                frame "Syringe" {
                  n125 = call "Initiate Syringe Home.vi"("error in (no error)"=w406) -> ("error out"=w405:errorcluster)  [unwired: 10 in]
                }
              }
              n126 = Concatenate Strings("Sample ", w398, " in Transfer" ("string")) -> (w386:string)
              n127 = Less?(x=0.01, y=w388) -> (x < y?=w379:bool)
              n128 = Select(t=w383, s=w379, f=Sample_Transfer_Container_Enumerator."None") -> (s? t:f=w380:T3)
              n129 = Select(t=w391, s=w379, f=Sample_Transfer_State_Enumerator."Polish") -> (s? t:f=w389:T2)
              n130 = Bundle By Name(cluster=w392, "Target Container"=w380) -> (w381:refnum<class "cRIO-CO2.lvclass">)
              n131 = Select(t=w386, s=w379, f="Sample pressure is too low to perform Transfer! -> Polish") -> (s? t:f=w384:string)
              n132 = call "Sample Transfer go for State.vi"("error in (no error)"=w396, "Sample Transfer State"=w389, "cRIO-CO2 in"=w381) -> ("error out"=w402:errorcluster, "cRIO-CO2 out"=w401:refnum<class "cRIO-CO2.lvclass">)  [unwired: 7 in]
            }
          }
        }
        frame "Home Syringe" {
          n133 = call "Sample Transfer go for State.vi"("error in (no error)"=w410, "State Timeout (Inf=no timeout )"=10.0, "Sample Transfer State"=Sample_Transfer_State_Enumerator."Start Freezer", "cRIO-CO2 in"=w413) -> ("error out"=w414:errorcluster, "cRIO-CO2 out"=w412:refnum<class "cRIO-CO2.lvclass">)  [unwired: 6 in]
        }
        frame "Start Freezer" {
          n134 = Unbundle By Name(w421) -> ("Target Container"=w427:T3)
          n135 = call "LN Master Valve.vi"("error in (no error)"=w419, "Action (Read State)"=enum16{"Read State", "Open", "Close"}."Open", "cRIO-CO2 in"=w421) -> ("error out"=w418:errorcluster, "cRIO-CO2 out"=w420:refnum<class "cRIO-CO2.lvclass">)  [unwired: 6 in, 1 out]
          n136 = call "Sample Transfer Set Freezer.vi"("Container"=w427, "error in (no error)"=w418, "ON/OFF(OFF)"=TRUE, "cRIO-CO2 in"=w420) -> ("error out"=w425:errorcluster, "Container Name String"=w422:string, "cRIO-CO2 out"=w424:refnum<class "cRIO-CO2.lvclass">)  [unwired: 5 in]
          n137 = Concatenate Strings("Start " ("String"), w422) -> (w423:string)
          n138 = call "Sample Transfer go for State.vi"("error in (no error)"=w425, "State Timeout (Inf=no timeout )"=1200.0, "Sample Transfer State"=Sample_Transfer_State_Enumerator."Freeze Target", "cRIO-CO2 in"=w424) -> ("error out"=w415:errorcluster, "cRIO-CO2 out"=w416:refnum<class "cRIO-CO2.lvclass">)  [unwired: 6 in]
        }
        frame "Freeze Target" {
          n139 = Unbundle By Name(w440) -> ("Target Container"=w435:T3)
          n140 = call "Sample Transfer Check Samples.vi"("error in (no error)"=w446, "cRIO-CO2 in"=w440) -> ("error out"=w444:errorcluster, "cRIO-CO2 out"=w445:refnum<class "cRIO-CO2.lvclass">, "Same Sample AND Target not Empty"=w442:bool)  [unwired: 5 in, 2 out]
          n141 = call "Is Conainer Frozen.vi"("Container"=w435, "error in (no error)"=w444, "cRIO-CO2 in"=w445) -> ("error out"=w437:errorcluster, "Is Frozen?"=w443:bool, "cRIO-CO2 out"=w439:refnum<class "cRIO-CO2.lvclass">)  [unwired: 5 in, 1 out]
          n142 = Not(x=w442) -> (.not. x?=w441:bool)
          n143 = Or(x=w441, y=w443) -> (x .or. y?=w434:bool)
          n144 = case shown="True" w434 {
            selector: w434 -> [w451 w452]
            tunnel: w439 -> [w449 w457]
            tunnel: [w449 w456] -> w438
            tunnel: w437 -> [w450 w455]
            tunnel: [w450 w454] -> w436
            tunnel: w435 -> [_ w453]
            tunnel: [w451 w452] -> w433
            frame False {
            }
            frame True {
              # "Open Target"
              n145 = call "Set Container.vi"("Container"=w453, "error in (no error)"=w455, "Open/Close (Close)"=w452, "cRIO-CO2 in"=w457) -> ("error out"=w454:errorcluster, "cRIO-CO2 out"=w456:refnum<class "cRIO-CO2.lvclass">)  [unwired: 6 in]
            }
          }
          n146 = call "Sample Transfer go for State.vi"("Really? (T)"=w433, "error in (no error)"=w436, "State Timeout (Inf=no timeout )"=1200.0, "Sample Transfer State"=Sample_Transfer_State_Enumerator."Crystalize", "cRIO-CO2 in"=w438) -> ("error out"=w447:errorcluster, "cRIO-CO2 out"=w448:refnum<class "cRIO-CO2.lvclass">)  [unwired: 5 in]
        }
        frame "Crystalize" {
          # "Stash threshold\nmBar"
          n147 = call "Preview Vacuum State.vi"("error in (no error)"=w477, "cRIO-CO2 in"=w481) -> ("error out"=w475:errorcluster, "State"=w463:T4, "cRIO-CO2 out"=w462:refnum<class "cRIO-CO2.lvclass">, "Raw Pressure"=w460:dbl)  [unwired: 3 in, 3 out]
          n148 = Unbundle By Name(w462) -> ("Target Container"=w464:T3, "Source Container"=w474:T3, "Transfer mBar"=w473:dbl, "Base Pressure"=w458:dbl)
          n149 = Subtract(x=w458, y=w460) -> (x-y=w459:dbl)
          n150 = call "Write Sample Transfer.mBar Transfered.vi"("mBar Transfered"=w459, "cRIO-CO2 in"=w462) -> ("cRIO-CO2 out"=w461:refnum<class "cRIO-CO2.lvclass">)  [unwired: 9 in]
          n151 = case shown="\"Pressure Rising\"" w463 {
            selector: w463 -> [_ _ w521 _]
            tunnel: w475 -> [w484 w508 w530 w567]
            tunnel: [w483 w498 w527 w568] -> w470
            tunnel: w461 -> [w483 w488 w529 w568]
            tunnel: w460 -> [_ w495 _ _]
            tunnel: [w484 w500 w526 w567] -> w471
            tunnel: w474 -> [_ w493 w528 _]
            tunnel: w473 -> [_ _ w519 _]
            tunnel: w478 -> [_ w507 w523 _]
            tunnel: [TRUE ("Timeout?") w507 w523 TRUE ("Timeout?")] -> w465
            tunnel: [w482 w506 w524 w565] -> w469
            tunnel: [w482 w502 "" ("f") w565] -> w468
            tunnel: "Crystalization timed out -> Abort" -> [_ w506 w524 _]
            tunnel: "Crystalization Complete" ("f") -> [_ w502 _ _]
            tunnel: w464 -> [_ w497 w522 _]
            tunnel: w459 -> [_ w486 w518 _]
            frame "Pressure Rising" {
              w482 = "Pressure in the Transfer Line is rising -> Abort."
              # "Pressure is rising and it's a good enough reason to Abort crystalization."
            }
            frame "Valley", "Low Valley" {
              # "Finalize mBar Transfered\nvalue"
              # "Stash to Storage only"
              n152 = Greater?(x=w495, y=5.0 ("Stash if more than")) -> (0:w496:bool)
              n153 = case shown="\"Storage 01\"..\"Storage 12\"" w493 {
                tunnel: [Sample_Transfer_State_Enumerator."Polish" ("t") Sample_Transfer_State_Enumerator."Initiate Stash" ("t")] -> w504
                frame Default {
                }
                frame "Storage 01".."Storage 12" {
                }
              }
              n154 = call "Write Sample Transfer.mBar Transfered.vi"("mBar Transfered"=w486, "cRIO-CO2 in"=w488) -> ("cRIO-CO2 out"=w487:refnum<class "cRIO-CO2.lvclass">)  [unwired: 9 in]
              n155 = Select(t=w504, s=w496, f=Sample_Transfer_State_Enumerator."Polish" ("Sample Transfer State")) -> (s? t:f=w494:T2)
              n156 = call "Read Sample Transfer Goal reached.vi"("cRIO-CO2 in"=w487) -> ("Goal reached"=w490:bool, "cRIO-CO2 out"=w491:refnum<class "cRIO-CO2.lvclass">)  [unwired: 9 in]
              n157 = call "Sample Transfer go for State.vi"("Restart Message (F)"=TRUE, "error in (no error)"=w508, "State Timeout (Inf=no timeout )"=10.0, "Sample Transfer State"=w494, "cRIO-CO2 in"=w491) -> ("error out"=w501:errorcluster, "cRIO-CO2 out"=w499:refnum<class "cRIO-CO2.lvclass">)  [unwired: 5 in]
              n158 = case shown="\"Polish\"" w494 {
                tunnel: w501 -> [w512 w517]
                tunnel: [w512 w514] -> w500
                tunnel: w499 -> [w511 w516]
                tunnel: [w511 w515] -> w498
                tunnel: w493 -> [_ _]
                tunnel: w497 -> [_ _]
                tunnel: w490 -> [_ _]
                frame Default {
                }
                frame "Polish" {
                  n159 = call "Set Turbo Valve.vi"("error in (no error)"=w517, "ON/OFF(OFF)"=TRUE, "cRIO-CO2 in"=w516) -> ("error out"=w514:errorcluster, "cRIO-CO2 out"=w515:refnum<class "cRIO-CO2.lvclass">)  [unwired: 7 in]
                }
              }
            }
            frame "Plateau", "Pressure Dropping" {
              n160 = Less?(x=w519, y=w518) -> (x < y?=w525:bool)
              n161 = case shown="True" w525 {
                tunnel: w530 -> [w535 w555]
                tunnel: w529 -> [w538 w549]
                tunnel: [w537 w550] -> w527
                tunnel: [w534 w551] -> w526
                tunnel: w528 -> [_ _]
                tunnel: w522 -> [_ w556]
                tunnel: w521 -> [_ w552]
                tunnel: w519 -> [w533 _]
                frame False {
                  n162 = Less?(x=w533, y=1000.0 ("x")) -> (x < y?=w531:bool)
                  n163 = case shown="True" w531 {
                    tunnel: w538 -> [w540 w546]
                    tunnel: [w540 w545] -> w537
                    tunnel: Time-Delay_Override_Options."Send next copy now" ("notification (Send next copy now)") -> [_ w544]
                    tunnel: w535 -> [w539 w543]
                    tunnel: [w539 w542] -> w534
                    frame False {
                    }
                    frame True {
                      n164 = call "Send Sample Transfer Notification.vi"("notification (Send next copy now)"=w544, "error in (no error)"=w543, "cRIO-CO2 in"=w546) -> ("error out"=w542:errorcluster, "cRIO-CO2 out"=w545:refnum<class "cRIO-CO2.lvclass">)  [unwired: 7 in]
                      n165 = Wait (ms)(milliseconds to wait=u32 50) -> ()  [unwired: 1 out]
                    }
                  }
                }
                frame True {
                  # "This will make vacuum state go\nFrom Dropping to Valley"
                  n166 = call "Write Sample Transfer Goal reached.vi"("Goal reached"=TRUE, "cRIO-CO2 in"=w549) -> ("cRIO-CO2 out"=w548:refnum<class "cRIO-CO2.lvclass">)  [unwired: 9 in]
                  n167 = case shown="\"Plateau\"" w552 {
                    tunnel: w555 -> [w559 w564]
                    tunnel: [w559 w563] -> w554
                    tunnel: w548 -> [w558 w562]
                    tunnel: [w558 w561] -> w553
                    frame Default {
                    }
                    frame "Plateau" {
                      # "Force Valley"
                      n168 = call "Sample Transfer Override Vacuum State.vi"("error in (no error)"=w564, "State (Plateau)"=Vacuum_State_Enumerator."Valley", "cRIO-CO2 in"=w562) -> ("error out"=w563:errorcluster, "cRIO-CO2 out"=w561:refnum<class "cRIO-CO2.lvclass">)  [unwired: 7 in]
                    }
                  }
                  n169 = call "Set Container.vi"("Container"=w556, "error in (no error)"=w554, "Open/Close (Close)"=FALSE, "cRIO-CO2 in"=w553) -> ("error out"=w551:errorcluster, "cRIO-CO2 out"=w550:refnum<class "cRIO-CO2.lvclass">)  [unwired: 6 in]
                }
              }
            }
            frame "Leak", "Unknown" {
              w565 = "Vacuum Leak or State Unknown -> Abort"
            }
          }
          n170 = Select(t=w469, s=w465, f=w468) -> (s? t:f=w476:string)
          n171 = call "Sample Transfer go for State.vi"("Really? (T)"=w465, "error in (no error)"=w471, "Sample Transfer State"=Sample_Transfer_State_Enumerator."Abort", "cRIO-CO2 in"=w470) -> ("error out"=w479:errorcluster, "cRIO-CO2 out"=w480:refnum<class "cRIO-CO2.lvclass">)  [unwired: 6 in]
        }
        frame "Initiate Stash" {
          # "Start Source Freezer"
          # "Close Target"
          # "Override State, Force Plateau"
          n172 = Unbundle By Name(w578) -> ("Target Container"=w576:T3, "Source Container"=w575:T3)
          n173 = call "Sample Transfer Override Vacuum State.vi"("error in (no error)"=w580, "State (Plateau)"=Vacuum_State_Enumerator."Plateau", "cRIO-CO2 in"=w578) -> ("error out"=w583:errorcluster, "cRIO-CO2 out"=w582:refnum<class "cRIO-CO2.lvclass">)  [unwired: 7 in]
          n174 = call "Sample Transfer Set Freezer.vi"("Container"=w575, "error in (no error)"=w583, "ON/OFF(OFF)"=TRUE, "cRIO-CO2 in"=w582) -> ("error out"=w585:errorcluster, "cRIO-CO2 out"=w586:refnum<class "cRIO-CO2.lvclass">)  [unwired: 5 in, 1 out]
          n175 = call "Set Container.vi"("Container"=w576, "error in (no error)"=w585, "Open/Close (Close)"=FALSE, "cRIO-CO2 in"=w586) -> ("error out"=w574:errorcluster, "cRIO-CO2 out"=w572:refnum<class "cRIO-CO2.lvclass">)  [unwired: 6 in]
          n176 = call "Sample Transfer go for State.vi"("error in (no error)"=w574, "State Timeout (Inf=no timeout )"=300.0, "Sample Transfer State"=Sample_Transfer_State_Enumerator."Stash", "cRIO-CO2 in"=w572) -> ("error out"=w573:errorcluster, "cRIO-CO2 out"=w571:refnum<class "cRIO-CO2.lvclass">)  [unwired: 6 in]
        }
        frame "Stash" {
          n177 = call "Preview Vacuum State.vi"("error in (no error)"=w608, "cRIO-CO2 in"=w612) -> ("error out"=w606:errorcluster, "State"=w605:T4, "Pressure (mBar)"=w600:dbl, "cRIO-CO2 out"=w604:refnum<class "cRIO-CO2.lvclass">)  [unwired: 3 in, 3 out]
          n178 = Unbundle By Name(w604) -> ("Target Container"=w593:T3, "Source Container"=w603:T3, "Transfer mBar"=w602:dbl, "Base Pressure"=w601:dbl)
          n179 = case shown="\"Pressure Dropping\"" w605 {
            tunnel: w606 -> [w624 w636 w637 w643 w649]
            tunnel: [w623 w634 w638 w644 w647] -> w588
            tunnel: w604 -> [w623 w635 w638 w644 w647]
            tunnel: w600 -> [_ _ _ _ _]
            tunnel: [w624 w633 w637 w643 w649] -> w592
            tunnel: w603 -> [_ _ _ _ _]
            tunnel: w602 -> [_ _ _ _ _]
            tunnel: w601 -> [_ _ _ _ _]
            tunnel: w609 -> [_ _ w640 _ _]
            tunnel: [TRUE ("Timeout?") FALSE ("Timeout?") w640 FALSE ("Timeout?") TRUE ("Timeout?")] -> w594
            tunnel: [w622 w631 w641 w646 "Vacuum Leak or State Unknown -> Abort"] -> w598
            tunnel: [w622 w632 _ _ _] -> w597
            tunnel: "Stashing timed out -> Abort" -> [_ w631 w641 w646 _]
            tunnel: "Stashing Complete" ("f") -> [_ w632 _ _ _]
            tunnel: w593 -> [w621 w629 w639 w645 w648]
            tunnel: [_ TRUE ("Open/Close (Close)") _ _ _] -> w589
            tunnel: [w621 w629 w639 w645 w648] -> w587
            frame "Pressure Rising" {
              w622 = "Pressure in the Transfer Line is rising -> Abort."
              # "Pressure is rising and it's a good enough reason to Abort."
            }
            frame "Valley", "Low Valley" {
              n180 = call "Sample Transfer go for State.vi"("error in (no error)"=w636, "State Timeout (Inf=no timeout )"=10.0, "Sample Transfer State"=Sample_Transfer_State_Enumerator."Polish", "cRIO-CO2 in"=w635) -> ("error out"=w633:errorcluster, "cRIO-CO2 out"=w634:refnum<class "cRIO-CO2.lvclass">)  [unwired: 6 in]
            }
            frame "Plateau" {
            }
            frame "Pressure Dropping" {
            }
            frame "Leak", "Unknown" {
            }
          }
          n181 = case shown="True" w589 {
            selector: w589 -> [_ w616]
            tunnel: w592 -> [w614 w620]
            tunnel: [w614 w619] -> w591
            tunnel: w588 -> [w613 w618]
            tunnel: [w613 w617] -> w590
            tunnel: w587 -> [_ w615]
            frame False {
            }
            frame True {
              n182 = call "Set Container.vi"("Container"=w615, "error in (no error)"=w620, "Open/Close (Close)"=w616, "cRIO-CO2 in"=w618) -> ("error out"=w619:errorcluster, "cRIO-CO2 out"=w617:refnum<class "cRIO-CO2.lvclass">)  [unwired: 6 in]
            }
          }
          n183 = Select(t=w598, s=w594, f=w597) -> (s? t:f=w607:string)
          n184 = call "Sample Transfer go for State.vi"("Really? (T)"=w594, "error in (no error)"=w591, "Sample Transfer State"=Sample_Transfer_State_Enumerator."Abort", "cRIO-CO2 in"=w590) -> ("error out"=w610:errorcluster, "cRIO-CO2 out"=w611:refnum<class "cRIO-CO2.lvclass">)  [unwired: 6 in]
        }
        frame "Polish" {
          n185 = call "Sample Transfer go for State.vi"("Really? (T)"=w654, "error in (no error)"=w653, "Sample Transfer State"=Sample_Transfer_State_Enumerator."Complete", "cRIO-CO2 in"=w652) -> ("error out"=w657:errorcluster, "cRIO-CO2 out"=w656:refnum<class "cRIO-CO2.lvclass">)  [unwired: 6 in]
        }
        frame "Stop Freezers" {
          # "This state is skipped for now.\nFreesers are stopped in the Complete State."
          n186 = Unbundle By Name(w668) -> ("Target Container"=w667:T3)
          n187 = call "Sample Transfer Set Freezer.vi"("Container"=w667, "error in (no error)"=w669, "ON/OFF(OFF)"=FALSE, "cRIO-CO2 in"=w668) -> ("error out"=w663:errorcluster, "Container Name String"=w664:string, "cRIO-CO2 out"=w661:refnum<class "cRIO-CO2.lvclass">)  [unwired: 5 in]
          n188 = Concatenate Strings("Stop " ("string"), w664) -> (w658:string)
          n189 = call "Sample Transfer go for State.vi"("error in (no error)"=w663, "Sample Transfer State"=Sample_Transfer_State_Enumerator."Complete", "cRIO-CO2 in"=w661) -> ("error out"=w662:errorcluster, "cRIO-CO2 out"=w660:refnum<class "cRIO-CO2.lvclass">)  [unwired: 7 in]
        }
        frame "Complete" {
          # "Finalize the transfer"
          n190 = call "Send Sample Transfer Notification.vi"("notification (Send next copy now)"=Time-Delay_Override_Options."Stop all further copies", "error in (no error)"=w689, "cRIO-CO2 in"=w680) -> ("error out"=w687:errorcluster, "cRIO-CO2 out"=w684:refnum<class "cRIO-CO2.lvclass">)  [unwired: 7 in]
          n191 = call "Sample Transfer Publish Progress.vi"("error in (no error)"=w687, "Progress"=u8 100, "cRIO-CO2 in"=w684) -> ("error out"=w673:errorcluster, "cRIO-CO2 out"=w670:refnum<class "cRIO-CO2.lvclass">)  [unwired: 7 in]
          n192 = call "Wait (wrapper).vi"("milliseconds to wait (200)"=u32 1000, "error in (no error)"=w673) -> ("error out"=w672:errorcluster)  [unwired: 9 in]
          n193 = call "Sample Transfer Close Source Container.vi"("error in (no error)"=w672, "cRIO-CO2 in"=w670) -> ("error out"=w674:errorcluster, "cRIO-CO2 out"=w675:refnum<class "cRIO-CO2.lvclass">)  [unwired: 8 in]
          n194 = call "Sample Transfer Close Target Container.vi"("error in (no error)"=w674, "cRIO-CO2 in"=w675) -> ("error out"=w677:errorcluster, "cRIO-CO2 out"=w676:refnum<class "cRIO-CO2.lvclass">)  [unwired: 8 in]
          n195 = call "Sample Transfer Stop Freezers and Blowers.vi"("error in (no error)"=w677, "cRIO-CO2 in"=w676) -> ("error out"=w678:errorcluster, "cRIO-CO2 out"=w679:refnum<class "cRIO-CO2.lvclass">)  [unwired: 8 in]
          n196 = Unbundle By Name(w679) -> ("Target Container"=w683:T3)
          n197 = case shown="\"Syringe\"" w683 {
            tunnel: w678 -> [w691 w696]
            tunnel: [w691 w700] -> w682
            tunnel: w679 -> [w690 w692]
            tunnel: [w690 w693] -> w681
            frame "None", Default {
            }
            frame "Syringe" {
              # "Initiate Sample Push"
              n198 = Unbundle By Name(w692) -> ("mBar Transfered"=w699:dbl, "Source Container"=w695:T3)
              n199 = call "Read Sample Transfer.Sample In Transfer.vi"("cRIO-CO2 in"=w692) -> ("Sample.lvclass"=w697:refnum<class "Sample.lvclass">, "cRIO-CO2 out"=w698:refnum<class "cRIO-CO2.lvclass">)  [unwired: 9 in]
              n200 = call "Write Sample Push.Sample.vi"("Sample.lvclass"=w697, "cRIO-CO2 in"=w698) -> ("cRIO-CO2 out"=w694:refnum<class "cRIO-CO2.lvclass">)  [unwired: 9 in]
              n201 = call "Initiate Sample Push.vi"("error in (no error)"=w696, "Source Storage (None)"=w695, "Sample mBar"=w699, "cRIO-CO2 in"=w694) -> ("error out"=w700:errorcluster, "cRIO-CO2 out"=w693:refnum<class "cRIO-CO2.lvclass">)  [unwired: 6 in]
            }
          }
        }
        frame "Abort" {
          n202 = call "Send Sample Transfer Notification.vi"("notification (Send next copy now)"=Time-Delay_Override_Options."Stop all further copies", "error in (no error)"=w713, "cRIO-CO2 in"=w711) -> ("error out"=w712:errorcluster, "cRIO-CO2 out"=w705:refnum<class "cRIO-CO2.lvclass">)  [unwired: 7 in]
          n203 = call "Sample Transfer Close All Containers.vi"("error in (no error)"=w712, "cRIO-CO2 in"=w705) -> ("error out"=w708:errorcluster, "cRIO-CO2 out"=w704:refnum<class "cRIO-CO2.lvclass">)  [unwired: 8 in]
          n204 = call "Set Turbo Valve.vi"("error in (no error)"=w708, "ON/OFF(OFF)"=FALSE, "cRIO-CO2 in"=w704) -> ("error out"=w706:errorcluster, "cRIO-CO2 out"=w703:refnum<class "cRIO-CO2.lvclass">)  [unwired: 7 in]
          n205 = call "Sample Transfer Stop Freezers and Blowers.vi"("error in (no error)"=w706, "cRIO-CO2 in"=w703) -> ("error out"=w701:errorcluster, "cRIO-CO2 out"=w702:refnum<class "cRIO-CO2.lvclass">)  [unwired: 8 in]
        }
      }
      n206 = case shown="Default" w17 {
        selector: w17 -> [w26 _]
        tunnel: w16 -> [w28 w30]
        tunnel: [w27 w30] -> w15
        tunnel: w12 -> [w25 w29]
        tunnel: [w24 w29] -> w14
        frame Default {
          # "Log message"
          n207 = call "Log Message.vi"("error in (no error)"=w28, "String"=w26, "Source Name"="Sample Transfer" ("Container Name String"), "cRIO-CO2 in"=w25) -> ("error out"=w27:errorcluster, "cRIO-CO2 out"=w24:refnum<class "cRIO-CO2.lvclass">)  [unwired: 6 in]
        }
        frame "" {
          # "Nothing to log"
        }
      }
    }
    frame Error {
    }
  }
  "error out" <- w9
  "cRIO-CO2 out" <- w7
  n208 = Get Date/Time In Seconds() -> (seconds since 1Jan1904=w6:timestamp)
  n209 = feedback-in #1(w6) -> ()
  n210 = feedback #1(w6) -> (w5:timestamp)
  n211 = To Extended Precision Float(1:w6) -> (0:w4:ext)
  n212 = To Extended Precision Float(1:w5) -> (0:w3:ext)
  n213 = Subtract(x=w4, y=w3) -> (x-y=w1:ext)
  "Waveform Chart" <- w1
  n214 = To Time Stamp(1:w1) -> (0:→"time stamp":timestamp)
